vi "Get Node by Path.vi"(8 "error in (no error)":errorcluster, 10 "System Definition Node Path":string, 11 "SysDef Ref":T1) -> (0 "error out":errorcluster, 2 "Node Ref":refnum<k24>, 3 "SysDef Ref Out":T1)   [LabVIEW 2019, in "Simple SysDef API.lvlib"]
uses:
  <userlib>/SimpleSysDef/Simple SysDef API.lvlib
  <userlib>/SimpleSysDef/_SubVIs/System Definition Reference.ctl
  NationalInstruments.VeriStand.SystemDefinitionAPI
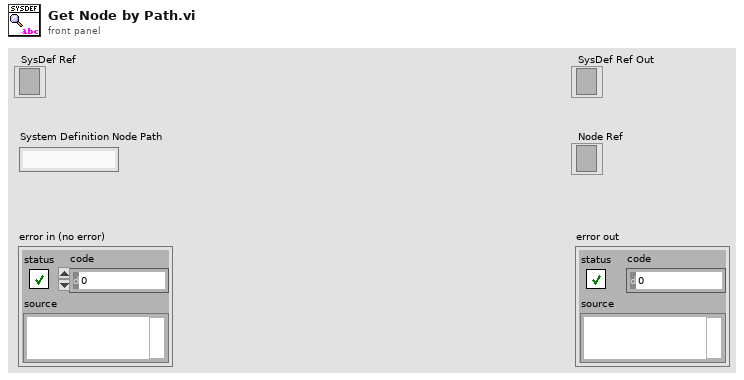
[diagram p1: front panel]
types:
  T1 = typedef "Simple SysDef API.lvlib/System Definition Reference.ctl" = refnum<k24>
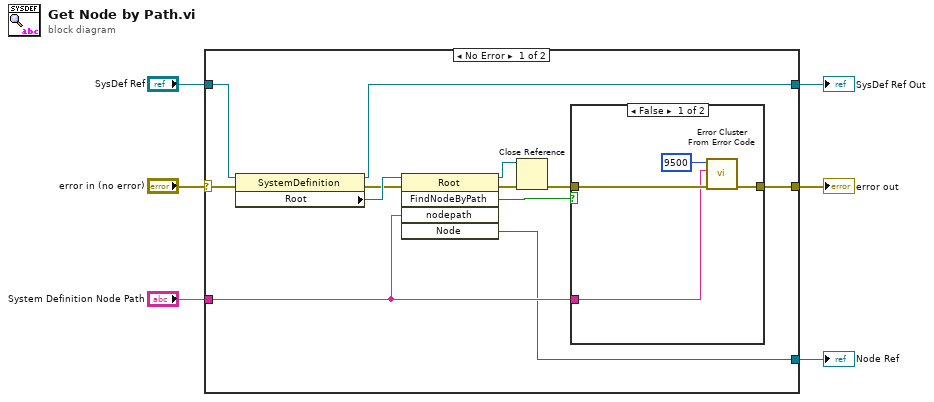
[diagram p0: block diagram]
diagram:
  n1 = case shown="No Error" "error in (no error)" {
    selector: "error in (no error)" -> [w18 w25]
    tunnel: [w9 w25] -> w5
    tunnel: "SysDef Ref" -> [w17 w24]
    tunnel: [w16 w24] -> w3
    tunnel: "System Definition Node Path" -> [w11 _]
    tunnel: [w7 _] -> w1
    frame No Error {
      n2 = property class="SystemDefinition"(reference=w17, error in=w18) -> (reference out=w16:T1, error out=w14:errorcluster, "Root"=w15:refnum<k24>)
      n3 = invoke class="Root" method="FindNodeByPath"(reference=w15, error in=w14, "nodepath"=w11) -> (reference out=w12:refnum<k24>, error out=w13:errorcluster, "FindNodeByPath"=w8:bool, "Node"=w7:refnum<k24>)  [unwired: 2 in, 1 out]
      n4 = Close Reference(reference=w12, error in (no error)=w13) -> (error out=w10:errorcluster)
      n5 = case shown="False" w8 {
        tunnel: w11 -> [w19 _]
        tunnel: w10 -> [w21 w23]
        tunnel: [w20 w23] -> w9
        frame False {
          n6 = call <userlib>:"Error Cluster From Error Code.vi"("error in (no error)"=w21, "error message (\"\")"=w19, "error code (0)"=9500 ("code")) -> ("error out"=w20:errorcluster)  [unwired: 6 in]
        }
        frame True {
        }
      }
    }
    frame Error {
    }
  }
  "SysDef Ref Out" <- w3
  "error out" <- w5
  "Node Ref" <- w1
